vi "Format JSON Array Text.vi"(8 "error in (no error)":errorcluster, 10 "Array of JSON Text":string[](array[string]), 11 "Pretty Print?":bool) -> (0 "error out":errorcluster, 3 "<JSON>":string)   [LabVIEW 2020, in "Library Commun.lvlib" / "JSON support.lvlib"]
uses:
  support/JSON support.lvlib
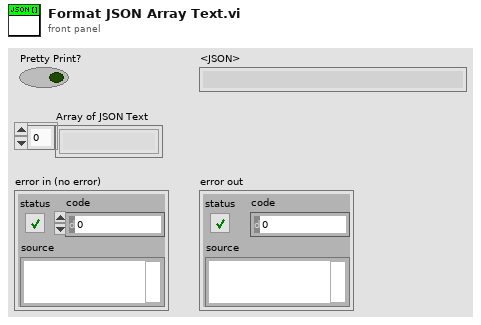
[diagram p1: front panel]
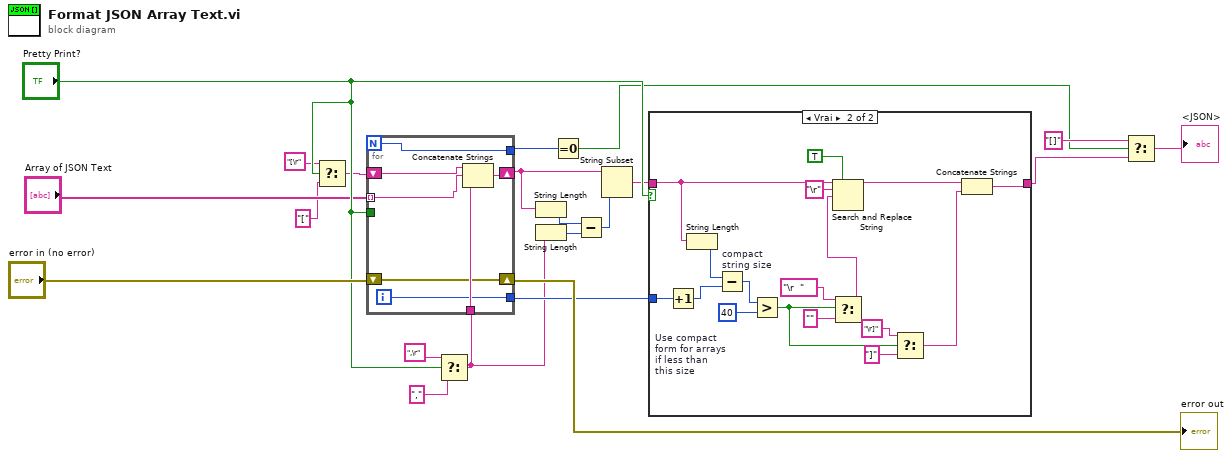
[diagram p0: block diagram]
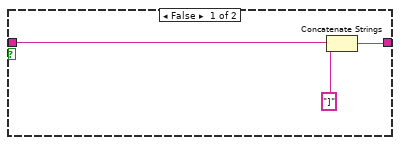
[diagram p2: hidden frame]
diagram:
  n1 = Select(t="[\r", s="Pretty Print?", f="[") -> (s? t:f=w9:string)
  n2 = Select(t=",\r" ("string"), s="Pretty Print?", f="," ("string")) -> (s? t:f=w14:string)
  n3 = for {
    N -> [w26]
    tunnel: "Array of JSON Text" -> [w23] mode=indexing
    shift-right: [w28] -> w5
    shift-left: w9 -> [w27]
    shift-right: [w22] -> w20
    shift-left: "error in (no error)" -> [w22]
    tunnel: "Pretty Print?" -> [_]
    tunnel: [w26] -> w2
    tunnel: w14 -> [w25]
    tunnel: [w24] -> w16
    i -> [w24]
    n4 = Concatenate Strings(w27, w23, w25) -> (w28:string)
  }
  "error out" <- w20
  n5 = String Length(string=w5) -> (length=w6:i32)
  n6 = String Length(string=w14) -> (length=w7:i32)
  n7 = Equal To 0?(x=w2) -> (x = 0?=w1:bool)
  n8 = Subtract(x=w6, y=w7) -> (x-y=w8:i32)
  n9 = String Subset(string=w5, length (rest)=w8) -> (substring=w11:string)  [unwired: 1 in]
  n10 = case shown="Vrai" "Pretty Print?" {
    tunnel: w11 -> [w29 w44]
    tunnel: [w30 w45] -> w15
    tunnel: w16 -> [_ w43]
    frame False {
      n11 = Concatenate Strings(w29, "]" ("substring (\"\")")) -> (w30:string)
    }
    frame True {
      w39 = 40  # Use compact form for arrays  if less than  this size
      n12 = Increment(x=w43) -> (x+1=w41:i32)
      n13 = String Length(string=w44) -> (length=w42:i32)
      n14 = Subtract "compact \nstring size"(x=w42, y=w41) -> (x-y=w40:i32)
      n15 = Greater?(x=w40, y=w39) -> (0:w35:bool)
      n16 = Select(t="\r  " ("search string"), s=w35, f="") -> (s? t:f=w36:string)
      n17 = Search and Replace String(replace all?=TRUE ("replace all? (F)"), input string=w44, search string="\r", replace string=w36) -> (result string=w46:string)  [unwired: 4 in, 3 out]
      n18 = Select(t="\r]" ("search string"), s=w35, f="]") -> (s? t:f=w32:string)
      n19 = Concatenate Strings(w46, w32) -> (w45:string)
    }
  }
  n20 = Select(t="[]", s=w1, f=w15) -> (s? t:f=→"<JSON>":string)
